vi "ConvertStringToClosedList.vi"(11 "Channel List":string) -> (3 "Channels Closed":bool[](array[boolean]))   [LabVIEW 2012, in "Keithley-7001.lvlib"]
uses:
  Keithley-7001.lvlib
panel:
  # "33"
  # "34"
  # "35"
  # "1"
  # "2"
  # "3"
  # "4"
  # "5"
  # "6"
  # "7"
  # "8"
  # "9"
  # "10"
  # "11"
  # "12"
  # "13"
  # "14"
  # "15"
  # "16"
  # "17"
  # "18"
  # "19"
  # "20"
  # "21"
  # "22"
  # "23"
  # "24"
  # "25"
  # "26"
  # "27"
  # "28"
  # "29"
  # "30"
  # "31"
  # "32"
  # "36"
  # "37"
  # "38"
  # "39"
  # "40"
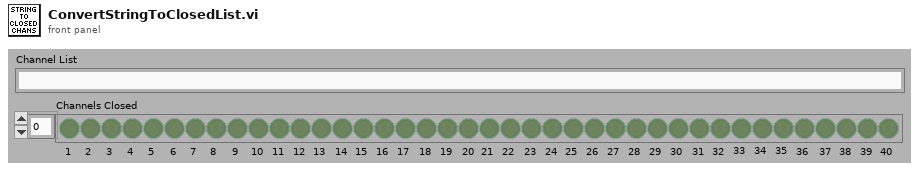
[diagram p1: front panel]
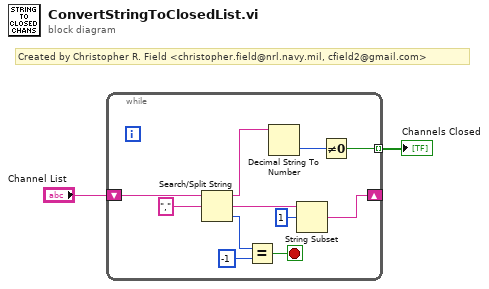
[diagram p0: block diagram]
diagram:
  # "Created by Christopher R. Field <christopher.field@nrl.navy.mil, cfield2@gmail.com>"
  n1 = while {
    shift-right: [w10] -> _
    shift-left: "Channel List" -> [w13]
    tunnel: [w3] -> w1 mode=indexing
    stop <- w4 stop-if-true
    n2 = Search/Split String(string=w13, search string/char (-)=",") -> (substring before match=w8:string, match + rest of string=w9:string, offset of match=w6:i32)  [unwired: 1 in]
    n3 = Equal?(x=w6, y=-1) -> (x = y?=w4:bool)
    n4 = Decimal String To Number(string=w8) -> (number=w7:i32)  [unwired: 2 in, 1 out]
    n5 = String Subset(string=w9, offset (0)=1) -> (substring=w10:string)  [unwired: 1 in]
    n6 = Not Equal To 0?(x=w7) -> (x != 0?=w3:bool)
  }
  "Channels Closed" <- w1
